vi "Read sensor 2.vi"(8 "error in (no error)":errorcluster, 10 "Sensor value in":dbl, 11 "VISA resource name in":refnum<visa-resource-name>) -> (0 "error out":errorcluster, 2 "Sensor value out":dbl, 3 "VISA resource name out":refnum<visa-resource-name>)   [LabVIEW 2020, in "Control de MaP.lvlib"]
uses:
  Control de MaP.lvlib
  Write--command.vi
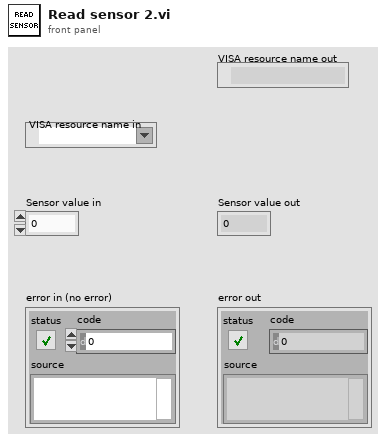
[diagram p1: front panel]
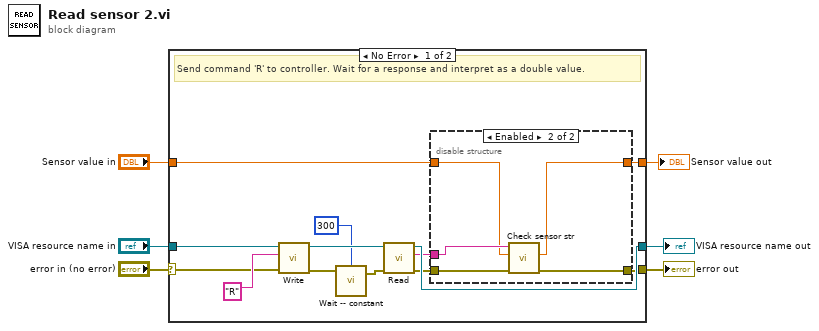
[diagram p0: block diagram]
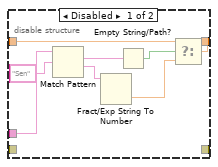
[diagram p2: hidden frame]
diagram:
  n1 = case shown="No Error" "error in (no error)" {
    selector: "error in (no error)" -> [w13 w34]
    tunnel: [w19 w35] -> w6
    tunnel: "Sensor value in" -> [w18 w35]
    tunnel: [w8 w34] -> w3
    tunnel: "VISA resource name in" -> [w12 w33]
    tunnel: [w11 w33] -> w1
    frame No Error {
      # "Send command 'R' to controller. Wait for a response and interpret as a double value."
      n2 = call-poly "Write.vi"("error in (no error)"=w13, "Command"="R", "VISA resource name"=w12) -> ("error out"=w15:errorcluster, "VISA resource name out"=w16:refnum<visa-resource-name>)  [unwired: 6 in, 1 out]
      n3 = call "Wait -- constant.vi"("wait (200 ms)"=u32 300 ("milliseconds\n to wait (200)"), "error in (no error)"=w15) -> ("error out"=w14:errorcluster)  [unwired: 3 in]
      n4 = call "Read.vi"("error in (no error)"=w14, "VISA resource name"=w16) -> ("error out"=w9:errorcluster, "Recibo de Datos"=w10:string, "VISA resource name out"=w11:refnum<visa-resource-name>)  [unwired: 6 in, 1 out]
      n5 = disable-structure shown="Enabled" {
        disable-tunnel: [w27 w28] -> w19
        disable-tunnel: w18 -> [w24 w29]
        disable-tunnel: w10 -> [w20 w30]
        disable-tunnel: w9 -> [_ w32]
        disable-tunnel: [_ w31] -> w8
        frame Disabled {
          n6 = Match Pattern(string=w20, regular expression="Sen") -> (match substring=w22:string, after substring=w25:string)  [unwired: 1 in, 2 out]
          n7 = Fract/Exp String To Number(string=w25) -> (number=w26:dbl)  [unwired: 3 in, 1 out]
          n8 = Empty String/Path?(string/path=w22) -> (empty?=w23:bool)
          n9 = Select(t=w24, s=w23, f=w26) -> (s? t:f=w27:dbl)
        }
        frame Enabled {
          n10 = call "Check sensor str.vi"("error in (no error)"=w32, "Sensor value in"=w29, "string"=w30) -> ("error out"=w31:errorcluster, "Sensor value out"=w28:dbl)  [unwired: 6 in]
        }
      }
    }
    frame Error {
    }
  }
  "Sensor value out" <- w6
  "error out" <- w3
  "VISA resource name out" <- w1
